vi "Download Data V.vi"(6 "year":i32, 7 "month":i32, 8 "error in (no error)":errorcluster, 9 "day":i32, 10 "hour":i32, 11 "minute":i32) -> (0 "error out":errorcluster, 3 "function return":i32)   [LabVIEW 2009, in "VantagePro.lvlib"]
doc: "DllAccess int _stdcall DownloadData_V(DateTimeStamp dateTimeStamp);"
uses:
  VantagePro.lvlib
  <userlib>/VantagePro/VantagePro.dll
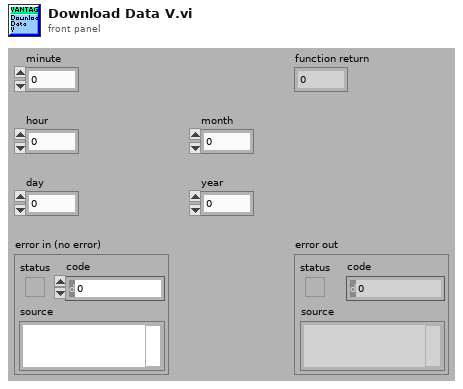
[diagram p1: front panel]
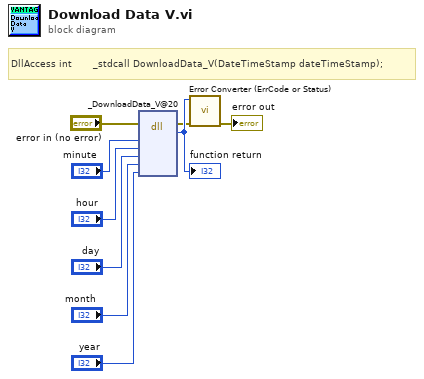
[diagram p0: block diagram]
diagram:
  # "DllAccess int       _stdcall DownloadData_V(DateTimeStamp dateTimeStamp);"
  n1 = dll-call lib="C:/Program Files/National Instruments/LabVIEW 2010/user.lib/VantagePro/VantagePro.*" fn="_DownloadData_V@20"(error in="error in (no error)", "minute"="minute", "hour"="hour", "day"="day", "month"="month", "year"="year") -> (error out=w2:errorcluster, w9:i32)  [unwired: 7 in, 1 out]
  "function return" <- w9
  n2 = call "Error Converter (ErrCode or Status).vi"("error in (no error)"=w2, "error code"=w9) -> ("error out"=→"error out":errorcluster)  [unwired: 9 in]
